vi "Parse Proposal.vi"(8 "error in":errorcluster, 9 "Parse from":enum16{"Proposal HTML:", "Proposal cluster"}(ring), 10 "Proposal Data":T3, 11 "Proposal document":path=path "C:/Users/l121767/Dropbox/Projects/FAIR/Project files/Proposal/National High Magnetic Field Laboratory - Users Program.html") -> (0 "error out":errorcluster, 3 "Puject  JSON":string)   [LabVIEW 2020]
uses:
  Utilities/iCalendar/Extract iCalendar String.ctl
  55103850-15ef-4a18-9388-7b0eadcdd449.vi
  <vilib>/JDP Science/JSONtext/Variant to JSON Text.vi
panel:
  in  "OSF Wiki":T1={"data"={"type"="wikis", "attributes"={"name"="", "content"=""}}}
  in  "OSF component":T2={"data"={"type"="nodes", "attributes"={"title"="", "description"="", "public"=FALSE, "category"=""}}}
  in  "OSF Project":T2={"data"={"type"="nodes", "attributes"={"title"="", "description"="", "public"=FALSE, "category"="project"}}}
  out "Proposal  title":string
  out "text":string
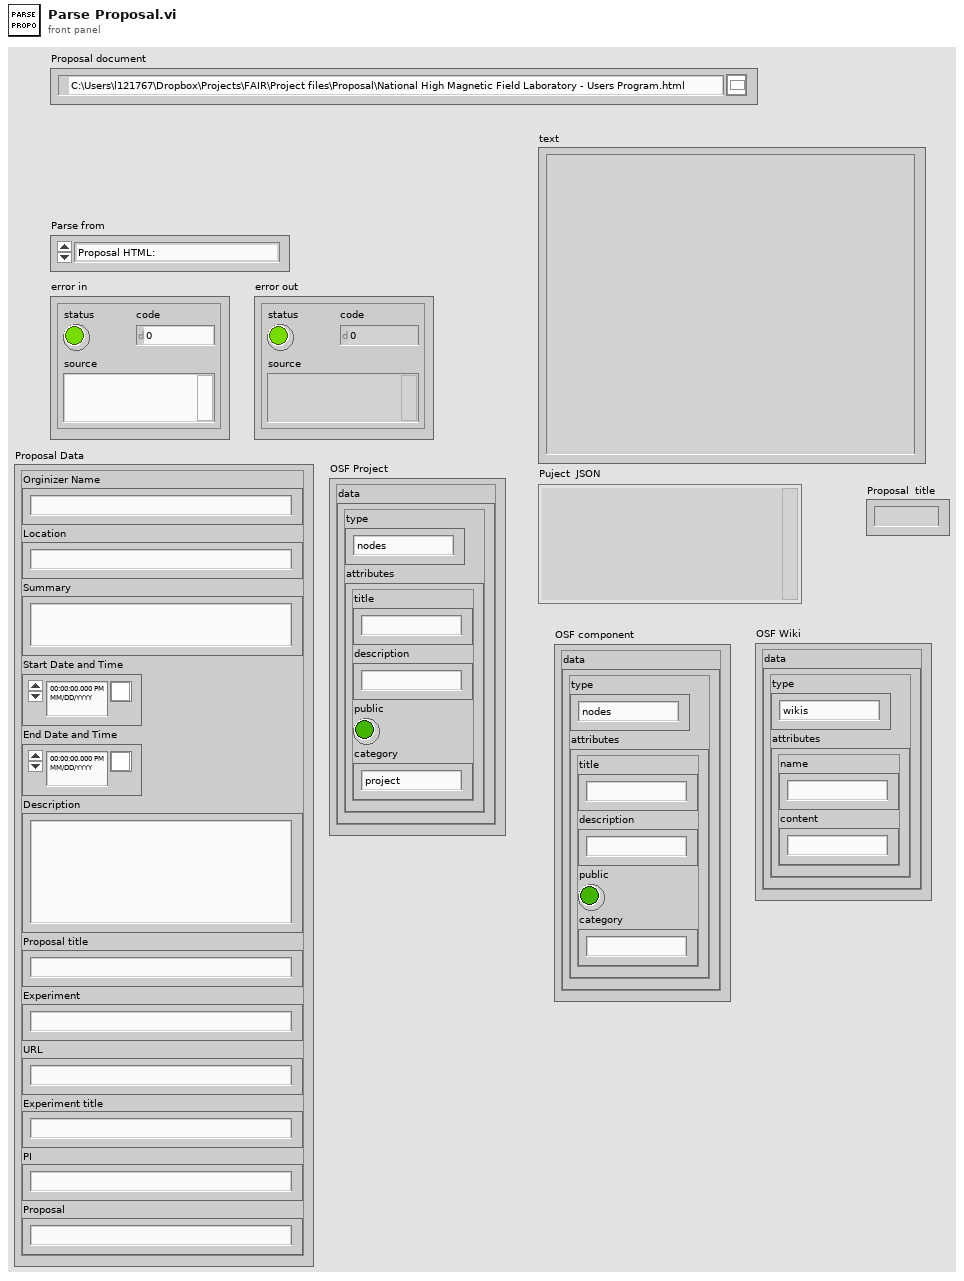
[diagram p1: front panel]
types:
  T1 = cluster{"data":cluster{"type":string, "attributes":cluster{"name":string, "content":string}}}
  T2 = cluster{"data":cluster{"type":string, "attributes":cluster{"title":string, "description":string, "public":bool, "category":string}}}
  T3 = typedef "Extract iCalendar String.ctl" = cluster{"Orginizer Name":string, "Location":string, "Summary":string, "Start Date and Time":timestamp, "End Date and Time":timestamp, "Description":string, "Proposal title":string, "Experiment":string, "URL":string, "Experiment title":string, "PI":string, "Proposal":string}
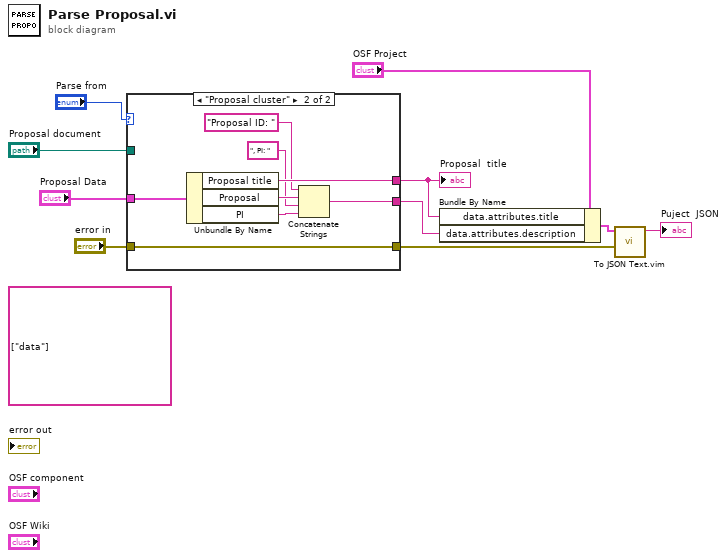
[diagram p0: block diagram]
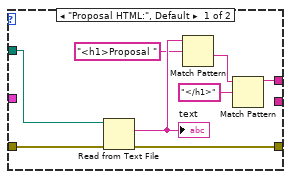
[diagram p2: hidden frame]
diagram:
  (unwired) string[] ["data"] ("Item Names")
  n1 = case shown="\"Proposal cluster\"" "Parse from" {
    tunnel: "Proposal document" -> [w18 _]
    tunnel: [w13 w25] -> w8
    tunnel: "error in" -> [w12 w24]
    tunnel: [w11 w24] -> w4
    tunnel: "Proposal Data" -> [_ w26]
    tunnel: [_ w23] -> w1
    frame "Proposal HTML:", Default {
      n2 = Read from Text File(file (use dialog)=w18, error in=w12) -> (text=w17:string, error out=w11:errorcluster)  [unwired: 2 in, 2 out]
      "text" <- w17
      n3 = Match Pattern(string=w17, regular expression="<h1>Proposal ") -> (after substring=w15:string)  [unwired: 1 in, 3 out]
      n4 = Match Pattern(string=w15, regular expression="</h1>") -> (before substring=w13:string)  [unwired: 1 in, 3 out]
    }
    frame "Proposal cluster" {
      n5 = Unbundle By Name(w26) -> ("Proposal title"=w25:string, "Proposal"=w20:string, "PI"=w22:string)
      n6 = Concatenate Strings("Proposal ID: " ("string"), w20, ", PI: " ("string"), w22) -> (w23:string)
    }
  }
  "Proposal  title" <- w8
  n7 = Bundle By Name(cluster="OSF Project", "data.attributes.title"=w8, "data.attributes.description"=w1) -> (w7:T2)
  n8 = call "To JSON Text.vim"("error in (no error)"=w4, "Anything"=w7) -> ("<JSON>"=→"Puject  JSON":string)  [unwired: 8 in, 1 out]
